vi "Module Top Level.vi"(8 "error in (no error)":errorcluster) -> (0 "error out":errorcluster)   [LabVIEW 2018, in "Error Handler.lvlib"]
doc: "This is the top level VI for this module. It uses a queue for communications and is stopped user a user event. The general architecture is similar to a simple queued message handler.\n\nThe VIs associated with this module are organized in a LabVIEW Library."
uses:
  Error Handler.lvlib
  Private Controls/Error Handler Data.ctl
panel:
  # "ERROR\nHANDLER"
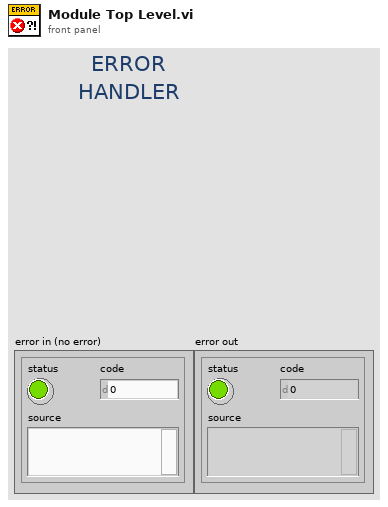
[diagram p1: front panel]
types:
  T1 = typedef "Error Handler.lvlib/Error Handler Data.ctl" = cluster{"Spare":bool}
  T2 = typedef "Error Handler.lvlib/Module Data.ctl" = cluster{"Data":variant, "Action":T3}
  T3 = typedef "Error Handler.lvlib/Module Action.ctl" = enum8{"Init", "Exit", "Controller Error", "UI1 Error", "UI2 Error", "UI3 Error", "File IO Error", "cRIO Error", "Calibration Error"}
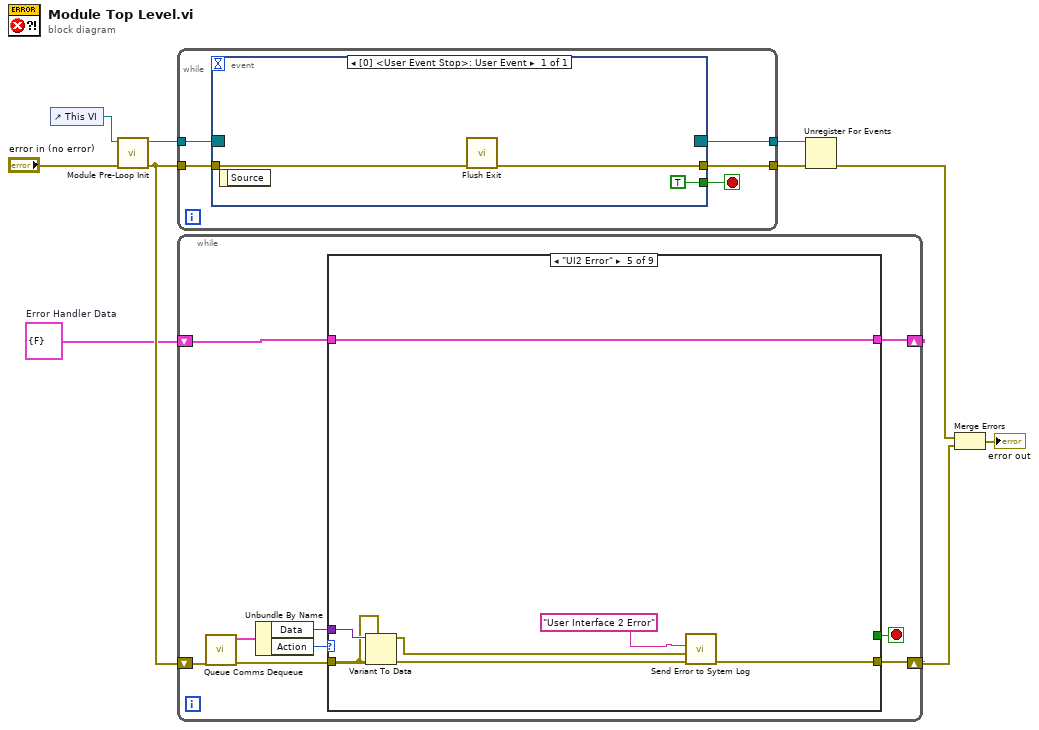
[diagram p0: block diagram]
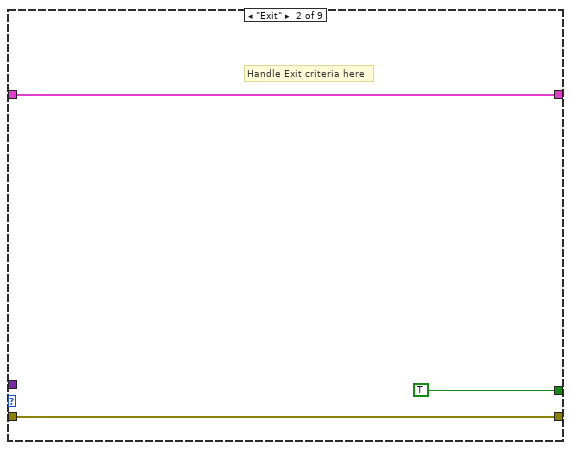
[diagram p3: hidden frame]
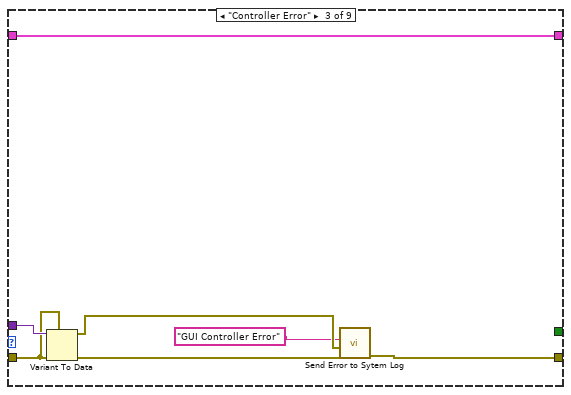
[diagram p4: hidden frame]
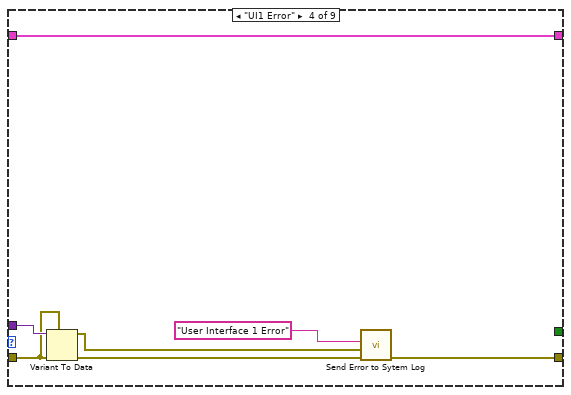
[diagram p5: hidden frame]
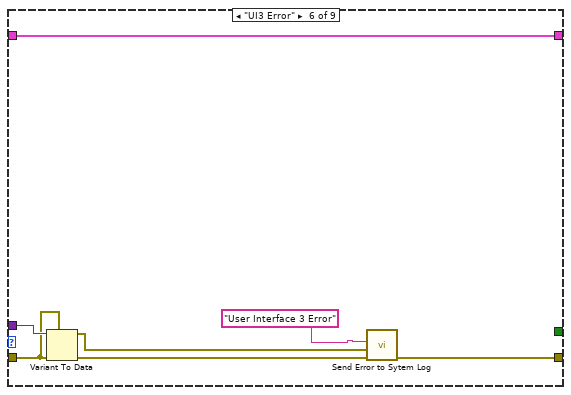
[diagram p6: hidden frame]
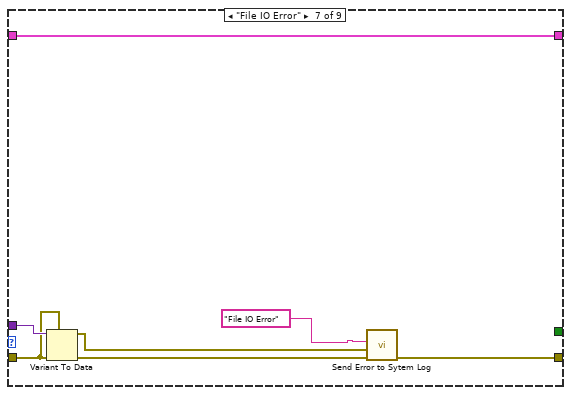
[diagram p7: hidden frame]
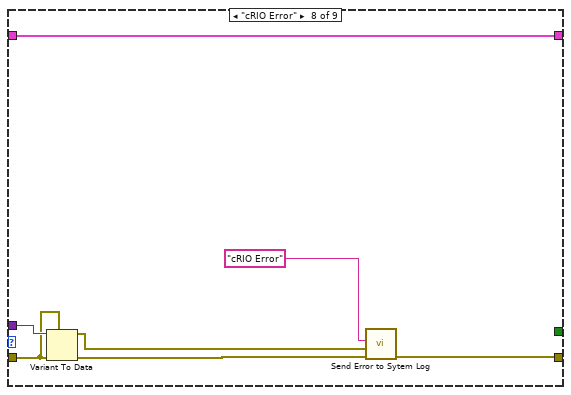
[diagram p8: hidden frame]
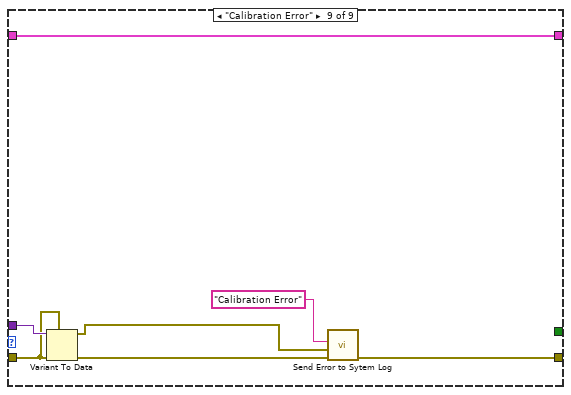
[diagram p9: hidden frame]
diagram:
  w1 = T1 {"Spare"=FALSE}  # Error Handler Data
  n1 = control-ref of="This VI"() -> (w10:refnum<vi>)
  n2 = call "Module Pre-Loop Init.vi"("error in (no error)"="error in (no error)", "Top Level VI Ref in"=w10) -> ("error out"=w2:errorcluster, "User Event Stop Ref"=w8:refnum<event-registration>)  [unwired: 8 in]
  n3 = while {
    tunnel: w8 -> [w15]
    tunnel: [w14] -> w6
    tunnel: w2 -> [w13]
    tunnel: [w11] -> w7
    stop <- w12 stop-if-true
    n4 = event shown="[0] <User Event Stop>: User Event" {
      selector: w15 -> [_]
      dyn-events: [_] -> w11
      timeout: _ -> [_]
      tunnel: [w16] -> w14
      tunnel: w13 -> [w17]
      tunnel: [TRUE] -> w12
      event User Event {
        n5 = event-data() -> ()  [unwired: 1 in, 1 out]
        n6 = call "Flush Exit.vi"("error in (no error)"=w17) -> ("error out"=w16:errorcluster)  [unwired: 10 in]
      }
    }
  }
  n7 = while {
    shift-right: [w19] -> w5
    shift-left: w2 -> [w20]
    shift-right: [w22] -> _
    shift-left: w1 -> [w21]
    stop <- w23 stop-if-true
    n8 = call "Queue Comms Dequeue.vi"("error in"=w20) -> ("error out"=w24:errorcluster, "element"=w27:T2)  [unwired: 9 in]
    n9 = Unbundle By Name(w27) -> ("Data"=w25:variant, "Action"=w26:T3)
    n10 = case shown="\"UI2 Error\"" w26 {
      tunnel: w25 -> [_ _ w39 w46 w53 w60 w67 w74 w81]
      tunnel: w24 -> [w29 w30 w38 w45 w52 w59 w66 w73 w80]
      tunnel: [w29 w30 w36 w43 w50 w57 w64 w71 w78] -> w19
      tunnel: [_ TRUE _ _ _ _ _ _ _] -> w23
      tunnel: [w28 w31 w35 w42 w49 w56 w62 w69 w76] -> w22
      tunnel: w21 -> [w28 w31 w35 w42 w49 w56 w62 w69 w76]
      frame "Init" {
      }
      frame "Exit" {
        # "Handle Exit criteria here"
      }
      frame "Controller Error" {
        n11 = Variant To Data(error in=w38, type=w38, Variant=w39) -> (data=w34:errorcluster, error out=w37:errorcluster)
        n12 = call "Send Error to Sytem Log.vi"("error in (no error)"=w37, "Error to Send"=w34, "Error Title or Message"="GUI Controller Error") -> ("error out"=w36:errorcluster)  [unwired: 8 in]
      }
      frame "UI1 Error" {
        n13 = Variant To Data(error in=w45, type=w45, Variant=w46) -> (data=w41:errorcluster, error out=w44:errorcluster)
        n14 = call "Send Error to Sytem Log.vi"("error in (no error)"=w44, "Error to Send"=w41, "Error Title or Message"="User Interface 1 Error") -> ("error out"=w43:errorcluster)  [unwired: 8 in]
      }
      frame "UI2 Error" {
        n15 = Variant To Data(error in=w52, type=w52, Variant=w53) -> (data=w48:errorcluster, error out=w51:errorcluster)
        n16 = call "Send Error to Sytem Log.vi"("error in (no error)"=w51, "Error to Send"=w48, "Error Title or Message"="User Interface 2 Error") -> ("error out"=w50:errorcluster)  [unwired: 8 in]
      }
      frame "UI3 Error" {
        n17 = Variant To Data(error in=w59, type=w59, Variant=w60) -> (data=w55:errorcluster, error out=w58:errorcluster)
        n18 = call "Send Error to Sytem Log.vi"("error in (no error)"=w58, "Error to Send"=w55, "Error Title or Message"="User Interface 3 Error") -> ("error out"=w57:errorcluster)  [unwired: 8 in]
      }
      frame "File IO Error" {
        n19 = Variant To Data(error in=w66, type=w66, Variant=w67) -> (data=w63:errorcluster, error out=w65:errorcluster)
        n20 = call "Send Error to Sytem Log.vi"("error in (no error)"=w65, "Error to Send"=w63, "Error Title or Message"="File IO Error") -> ("error out"=w64:errorcluster)  [unwired: 8 in]
      }
      frame "cRIO Error" {
        n21 = Variant To Data(error in=w73, type=w73, Variant=w74) -> (data=w70:errorcluster, error out=w72:errorcluster)
        n22 = call "Send Error to Sytem Log.vi"("error in (no error)"=w72, "Error to Send"=w70, "Error Title or Message"="cRIO Error") -> ("error out"=w71:errorcluster)  [unwired: 8 in]
      }
      frame "Calibration Error" {
        n23 = Variant To Data(error in=w80, type=w80, Variant=w81) -> (data=w77:errorcluster, error out=w79:errorcluster)
        n24 = call "Send Error to Sytem Log.vi"("error in (no error)"=w79, "Error to Send"=w77, "Error Title or Message"="Calibration Error") -> ("error out"=w78:errorcluster)  [unwired: 8 in]
      }
    }
  }
  n25 = Unregister For Events(event registration refnum=w7, error in=w6) -> (error out=w3:errorcluster)
  n26 = Merge Errors(w3, w5) -> (→"error out":errorcluster)
